vi "Bury All Target.vi"() -> ()   [LabVIEW 2018, in "Tests.lvlib" / "Bookmark Manager.lvlib" / "Unit.lvlib"]
uses:
  Unit.lvlib
panel:
  in  "Input 3":bool[](array[boolean])=[FALSE, FALSE, FALSE, TRUE, FALSE, FALSE]
  out "Any? 3":bool
  in  "Input 2":bool[](array[boolean])=[FALSE, FALSE, FALSE, TRUE, FALSE, FALSE]
  out "Any? 2":bool
  in  "Input 1":bool[](array[boolean])=[FALSE, FALSE, FALSE, TRUE, FALSE, FALSE]
  out "Any? 1":bool
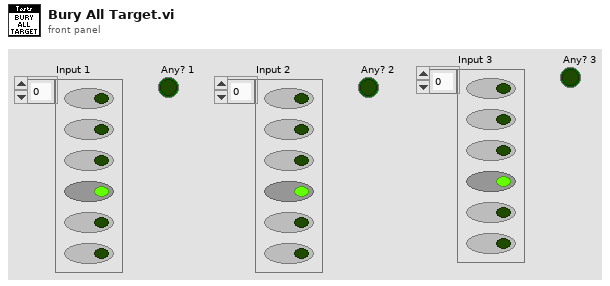
[diagram p1: front panel]
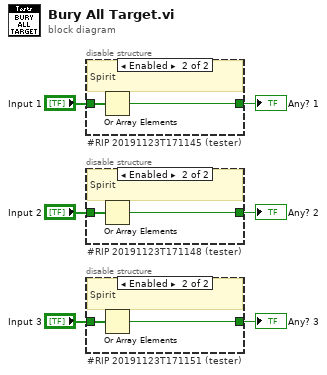
[diagram p0: block diagram]
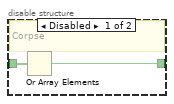
[diagram p2: hidden frame]
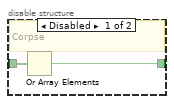
[diagram p3: hidden frame]
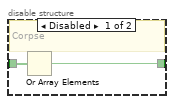
[diagram p4: hidden frame]
diagram:
  n1 = disable-structure "#RIP 20191123T171145 (tester)" shown="Enabled" {
    disable-tunnel: "Input 1" -> [w8 w10]
    disable-tunnel: [w7 w9] -> w5
    frame Disabled {
      # "Corpse"
      n2 = Or Array Elements(Boolean array=w8) -> (logical OR=w7:bool)
    }
    frame Enabled {
      # "Spirit"
      n3 = Or Array Elements(Boolean array=w10) -> (logical OR=w9:bool)
    }
  }
  "Any? 1" <- w5
  n4 = disable-structure "#RIP 20191123T171148 (tester)" shown="Enabled" {
    disable-tunnel: "Input 2" -> [w12 w14]
    disable-tunnel: [w11 w13] -> w3
    frame Disabled {
      # "Corpse"
      n5 = Or Array Elements(Boolean array=w12) -> (logical OR=w11:bool)
    }
    frame Enabled {
      # "Spirit"
      n6 = Or Array Elements(Boolean array=w14) -> (logical OR=w13:bool)
    }
  }
  "Any? 2" <- w3
  n7 = disable-structure "#RIP 20191123T171151 (tester)" shown="Enabled" {
    disable-tunnel: "Input 3" -> [w16 w18]
    disable-tunnel: [w15 w17] -> w1
    frame Disabled {
      # "Corpse"
      n8 = Or Array Elements(Boolean array=w16) -> (logical OR=w15:bool)
    }
    frame Enabled {
      # "Spirit"
      n9 = Or Array Elements(Boolean array=w18) -> (logical OR=w17:bool)
    }
  }
  "Any? 3" <- w1
